vi "DetectMultiBusPCIDGsHW.vi"(8 "error in (no error)":errorcluster, 11 "BME_DG_System in":refnum<class "BME_DG_System.lvclass">) -> (0 "error out":errorcluster, 1 "Errors":errorcluster[](array[cluster]), 2 "InstalledDGs":T1[](array[typedef]), 3 "BME_DG_System out":refnum<class "BME_DG_System.lvclass">, 5 "#DGs":i32)   [LabVIEW 2009, in "POLARIS BME DG.lvlib" / "BME_DG_System.lvclass"]
doc: "VI gets number of DG installed in computer by calling DLL DetectPCIDalayGenerators.\nThen VI aquire information about DG type, master or slave, bus number and slot number.\n\nThis VI is used for DG system configuration. \n\nATTENTION: it dactivates and resets all DGs. Make sure, you plant will not be damage by this. \n\n\n\n---------------\n\nauthor: Alexander Kessler, Helmholtz-Institut-Jena \nmaintainer: Alexander Kessler: alexander.kessler@uni-jena.de\n\n\nLicense Agreement for this software:\n\nCopyright (C)\nHelmholtz-Institut-Jena\nFröbelsteg 3\n07743 Jena\nGermany\n\nContact: alexander.kessler@uni-jena.de\n\nThis program is free software; you can redistribute it and/or modify it under the terms of the GNU General Public License as published by the Free Software Foundation; either version 2 of the license, or (at your option) any later version.\n\nThis program is distributed in the hope that it will be useful, but WITHOUT ANY WARRANTY; without even the implied warranty of MERCHANTABILITY or FITNESS FOR A PARTICULAR PURPOSE. See the GNU General License for more details (http://www.gnu.org)."
uses:
  BME_DG_System.lvclass
  DetectDG.ctl
  POLARIS BME DG.lvlib
panel:
  in  "?":T1
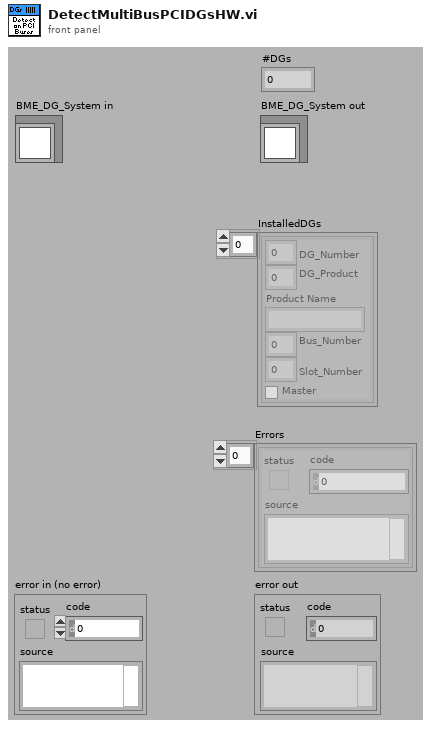
[diagram p1: front panel]
types:
  T1 = typedef "POLARIS BME DG.lvlib/DetectDG.ctl" = cluster{"DG_Number":i32, "DG_Product":i32, "Product Name":string, "Bus_Number":i32, "Slot_Number":i32, "Master":bool}
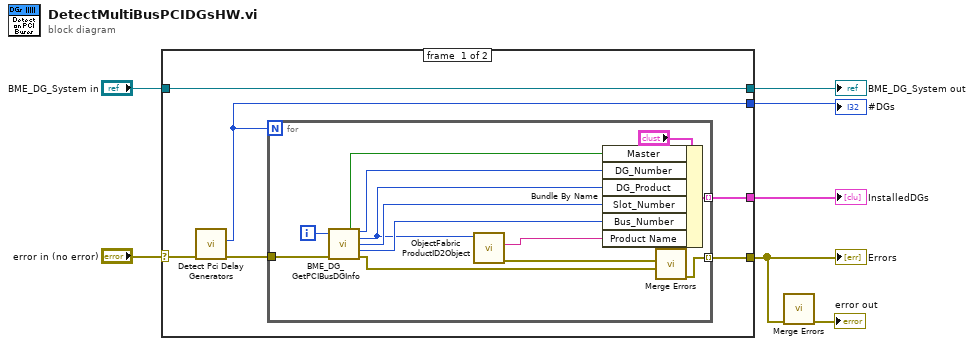
[diagram p0: block diagram]
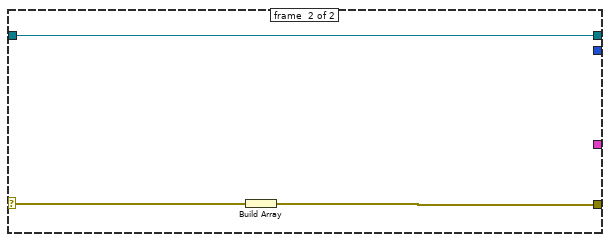
[diagram p2: hidden frame]
diagram:
  n1 = case shown="No Error" "error in (no error)" {
    selector: "error in (no error)" -> [w12 w29]
    tunnel: [w10 w27] -> w3
    tunnel: [w13 w28] -> w5
    tunnel: "BME_DG_System in" -> [w13 w28]
    tunnel: [w9 _] -> w4
    tunnel: [w8 _] -> w1
    frame #0 {
      n2 = call "Detect Pci Delay Generators.vi"("error in (no error)"=w12) -> ("error out"=w11:errorcluster, "Number of Generators"=w8:i32)  [unwired: 8 in, 1 out]
      n3 = for {
        N: w8 -> [_]
        tunnel: w11 -> [w25]
        tunnel: [w18] -> w10 mode=indexing
        tunnel: [w20] -> w9 mode=indexing
        i -> [w26]
        n4 = call "BME_DG_GetPCIBusDGInfo.vi"("DG_Number in"=w26, "error in (no error)"=w25) -> ("Master"=w17:bool, "DG_Number out"=w24:i32, "DG_Product"=w19:i32, "SlotNumber"=w23:i32, "Bus_Number"=w22:i32, "error out"=w14:errorcluster)  [unwired: 8 in]
        n5 = call "ObjectFabric ProductID2Object.vi"("DG_Product"=w19) -> ("error out"=w15:errorcluster, "ProductName"=w16:string)  [unwired: 8 in, 1 out]
        n6 = Bundle By Name(cluster="?", "Master"=w17, "DG_Number"=w24, "DG_Product"=w19, "Slot_Number"=w23, "Bus_Number"=w22, "Product Name"=w16) -> (w20:T1)
        n7 = call <vilib>:"Merge Errors.vi"("error in 3 (no error)"=w14, "error in 2 (no error)"=w15) -> ("error out"=w18:errorcluster)  [unwired: 5 in]
      }
    }
    frame #1 {
      n8 = Build Array(w29) -> (w27:errorcluster[])
    }
  }
  "BME_DG_System out" <- w5
  "Errors" <- w3
  "InstalledDGs" <- w4
  "#DGs" <- w1
  n9 = call <vilib>:"Merge Errors.vi"("error array in"=w3) -> ("error out"=→"error out":errorcluster)  [unwired: 6 in]
